vi "testGetSenMfromFile.vi"(8 "error in (no error)":errorcluster) -> (0 "error out":errorcluster)   [LabVIEW 2016]
doc: "Test to get the sensitivity matrix M from txt file."
uses:
  <vilib>/addons/_JKI Toolkits/Caraya/classes/Assert/Assert.lvclass
  <vilib>/addons/_JKI Toolkits/Caraya/classes/Test/Test.lvclass
  MatOper/MatOper.lvclass
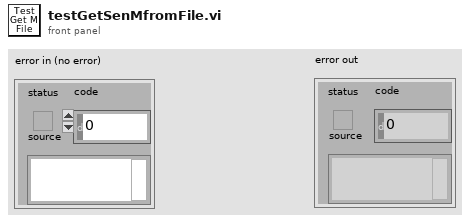
[diagram p1: front panel]
types:
  T1 = cluster{"Num of Field":i32, "Num of Zk":i32, "Num of DOF":i32}
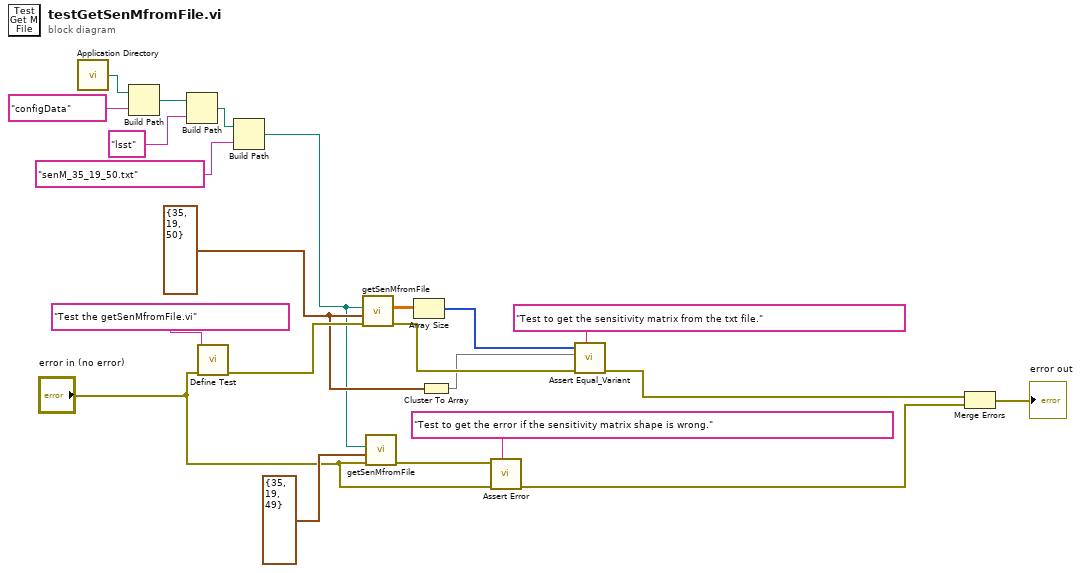
[diagram p0: block diagram]
diagram:
  w16 = T1 {"Num of Field"=35, "Num of Zk"=19, "Num of DOF"=50} ("Sensitivity Matrix Shape")
  n1 = call <vilib>:"Application Directory.vi"() -> ("Application Directory"=w7:path)
  n2 = Build Path(base path=w7, name or relative path="configData") -> (appended path=w5:path)
  n3 = Build Path(base path=w5, name or relative path="lsst") -> (appended path=w3:path)
  n4 = call <vilib>:"Define Test.vi"("error in (no error)"="error in (no error)", "Label (VI Title)"="Test the getSenMfromFile.vi") -> ("error out"=w20:errorcluster)  [unwired: 9 in]
  n5 = Build Path(base path=w3, name or relative path="senM_35_19_50.txt") -> (appended path=w1:path)
  n6 = call "getSenMfromFile.vi"("error in (no error)"=w20, "Sensitivity Matrix Shape"=w16, "Path"=w1) -> ("error out"=w19:errorcluster, "Sensitivity Matrix"=w18:dbl[][][])  [unwired: 6 in, 1 out]
  n7 = call "getSenMfromFile.vi"("error in (no error)"="error in (no error)", "Sensitivity Matrix Shape"=T1 {"Num of Field"=35, "Num of Zk"=19, "Num of DOF"=49}, "Path"=w1) -> ("error out"=w13:errorcluster)  [unwired: 6 in, 2 out]
  n8 = Array Size(array=w18) -> (size(s)=w17:i32[])
  n9 = Cluster To Array(cluster=w16) -> (array=w15:i32[])
  n10 = call <vilib>:"Assert Error.vi"("Label"="Test to get the error if the sensitivity matrix shape is wrong.", "error in (no error)"="error in (no error)", "Error?"=w13) -> ("error out"=w8:errorcluster)  [unwired: 8 in]
  n11 = call <vilib>:"Assert Equal_Variant.vi"("Label"="Test to get the sensitivity matrix from the txt file.", "error in (no error)"=w19, "Y"=w15, "X"=w17) -> ("error out"=w9:errorcluster)  [unwired: 7 in]
  n12 = Merge Errors(w9, w8) -> (→"error out":errorcluster)
